vi "TestScanForDevices.vi"(8 "error in (no error)":errorcluster) -> (0 "error out":errorcluster)   [LabVIEW 2019]
uses:
  <vilib>/addons/_JKI Toolkits/Caraya/classes/Test/Test.lvclass
  <vilib>/addons/_JKI Toolkits/Caraya/classes/Assert/Assert.lvclass
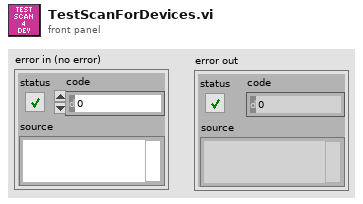
[diagram p1: front panel]
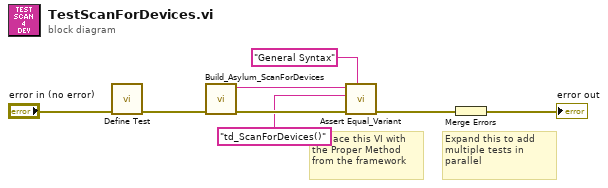
[diagram p0: block diagram]
diagram:
  # "Expand this to add multiple tests in parallel"
  # "Replace this VI with the Proper Method from the framework"
  n1 = call <vilib>:"Define Test.vi"("error in (no error)"="error in (no error)") -> ("error out"=w6:errorcluster)  [unwired: 10 in]
  n2 = call "Build_Asylum_ScanForDevices.vi"("error in (no error)"=w6) -> ("error out"=w5:errorcluster, "Command"=w3:string)  [unwired: 9 in]
  n3 = call <vilib>:"Assert Equal_Variant.vi"("Label"="General Syntax", "error in (no error)"=w5, "Y"="td_ScanForDevices()", "X"=w3) -> ("error out"=w4:errorcluster)  [unwired: 7 in]
  n4 = Merge Errors(w4) -> (→"error out":errorcluster)
